vi "Get_SubPaneVIRef.vi"(8 "error in (no error)":errorcluster, 10 "SubPanelName":string="SubPanel", 11 "CtlLookup In":T1) -> (0 "error out":errorcluster, 1 "SubPanelRef":refnum<vi>, 2 "VI out":refnum<vi>, 3 "CtlLookup Out":T1)   [LabVIEW 2020, in "CtlReferences.lvlib" / "CtlReferences.lvclass"]
doc: "This VI gets the reference to subpanel, and associated VI"
uses:
  CtlReferences.lvclass
  TypeDefs/CtlLookup.ctl
  GetControlRef/GetControl_SubPanel.vi
  GetCtlRef.vi
  Error_ToSpecificClass.vi
  CtlReferences.lvclass/CtlReferences.ctl
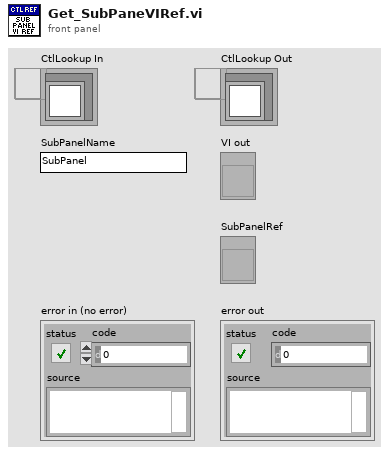
[diagram p1: front panel]
types:
  T1 = typedef "CtlReferences.lvlib/CtlReferences.lvclass/CtlLookup.ctl" = refnum<data-value>
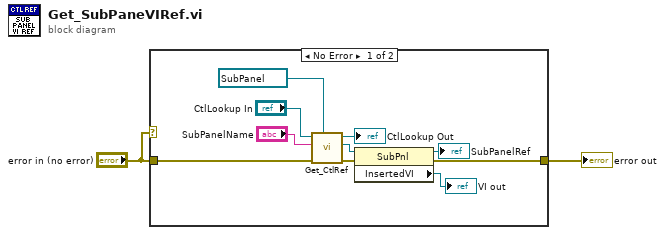
[diagram p0: block diagram]
diagram:
  n1 = case shown="No Error" "error in (no error)" {
    tunnel: "error in (no error)" -> [w11 w13]
    tunnel: [w4 w13] -> w2
    frame No Error {
      n2 = call-poly "Get_CtlRef.vi"("Control Class"=refnum<vi> refnum, "error in (no error)"=w11, "Control Label"="SubPanelName", "CtlLookup In"="CtlLookup In") -> ("error out"=w8:errorcluster, "Reference Out"=w7:refnum<vi>, "CtlLookup Out"=→"CtlLookup Out":T1)  [unwired: 5 in]
      n3 = property class="SubPnl"(reference=w7, error in=w8) -> (reference out=→"SubPanelRef":refnum<vi>, error out=w4:errorcluster, "InsertedVI"=→"VI out":refnum<vi>)
    }
    frame Error {
    }
  }
  "error out" <- w2
